vi "Inverse Kinematics Test.vi"() -> ()   [LabVIEW 2020]
panel:
  out "XY Graph":cluster{dbl[], dbl[]}[](graph)
  in  "Target Delta":dbl[](array[numeric]) format="%.2f"
  in  "Radii":T1 {"R4" format="%.2f"; "R3" format="%.2f"; "R2" format="%.2f"; "R1" format="%.2f"}
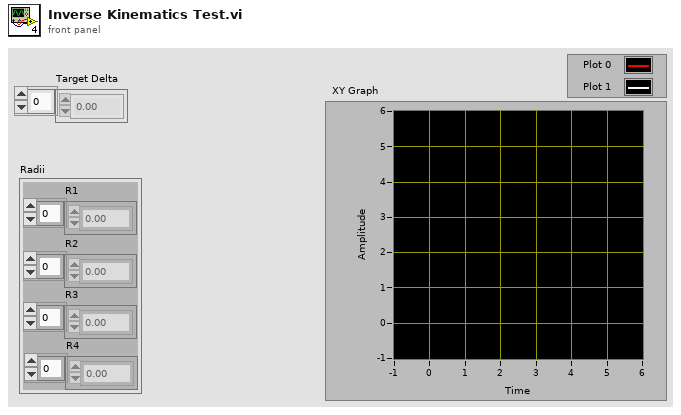
[diagram p1: front panel]
types:
  T1 = cluster{"R1":dbl[], "R2":dbl[], "R3":dbl[], "R4":dbl[]}
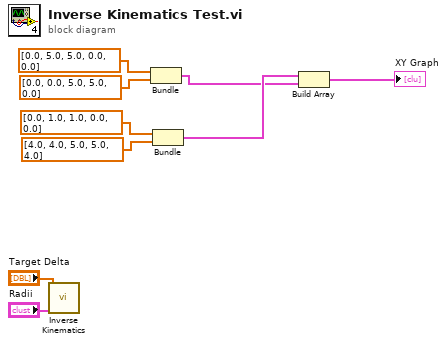
[diagram p0: block diagram]
diagram:
  n1 = call "Inverse Kinematics.vi"("Radii"="Radii", "Target Delta"="Target Delta") -> ()  [unwired: 6 in, 4 out]
  n2 = Bundle(dbl[] [0.0, 5.0, 5.0, 0.0, 0.0], dbl[] [0.0, 0.0, 5.0, 5.0, 0.0]) -> (w1:cluster{dbl[], dbl[]})  [unwired: 1 in]
  n3 = Bundle(dbl[] [0.0, 1.0, 1.0, 0.0, 0.0], dbl[] [4.0, 4.0, 5.0, 5.0, 4.0]) -> (w2:cluster{dbl[], dbl[]})  [unwired: 1 in]
  n4 = Build Array(w2, w1) -> (→"XY Graph":cluster{dbl[], dbl[]}[])
